vi "记录表与报警表-内容.vi"(10 "列数":u32, 11 "总大小":i32) -> (3 "列首":string[](array[string]))   [LabVIEW 2017]
panel:
  in  "列首 3":string[](array[string])
  in  "内容":string[](array[string])
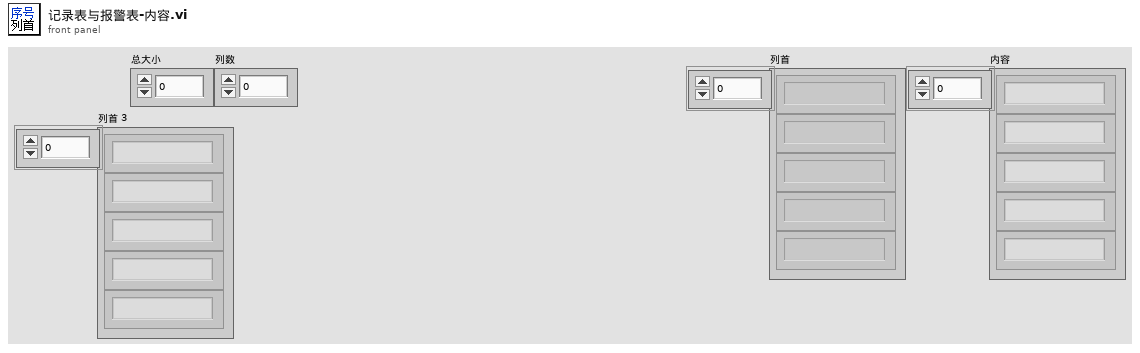
[diagram p1: front panel]
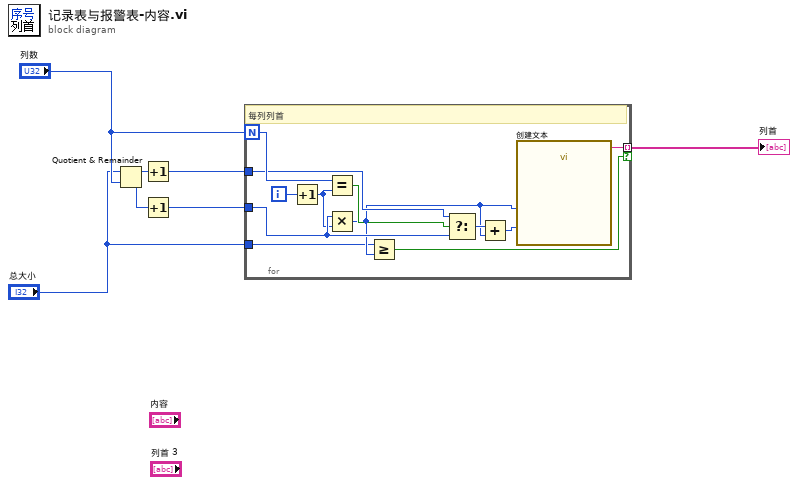
[diagram p0: block diagram]
diagram:
  n1 = Quotient & Remainder(x="总大小", y="列数") -> (x-y*floor(x/y)=w5:u32, floor(x/y)=w6:u32)
  n2 = Increment(x=w5) -> (x+1=w1:u32)
  n3 = Increment(x=w6) -> (x+1=w2:u32)
  n4 = for {
    N: "列数" -> [w19]
    tunnel: w2 -> [w13]
    tunnel: w1 -> [w17]
    tunnel: [w14] -> w4 mode=indexing if=w10
    tunnel: "总大小" -> [w11]
    i -> [w9]
    # "每列列首"
    n5 = Increment(x=w9) -> (x+1=w8:i32)
    n6 = Equal?(x=w19, y=w8) -> (x = y?=w18:bool)
    n7 = Multiply(x=w13, y=w8) -> (x*y=w12:u32)
    n8 = Greater Or Equal?(x=w11, y=w12) -> (x >= y?=w10:bool)
    n9 = Select(t=w17, s=w18, f=w13) -> (s? t:f=w16:u32)
    n10 = Add(x=w16, y=w12) -> (x+y=w15:u32)
    n11 = call "创建文本"("起始编号"=w12, "截止编号"=w15) -> ("Result"=w14:string)  [unwired: 12 in, 1 out]
  }
  "列首" <- w4
